vi "RampFunction.vi"(10 "Max Rate":dbl=1.0, 11 "Input":dbl(slide) scale=0.0..10.0) -> (3 "Output":dbl)   [LabVIEW 2016]
panel:
  # "r"
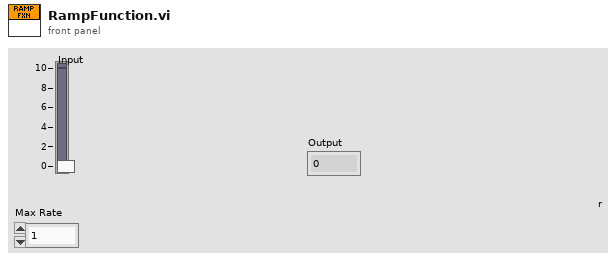
[diagram p1: front panel]
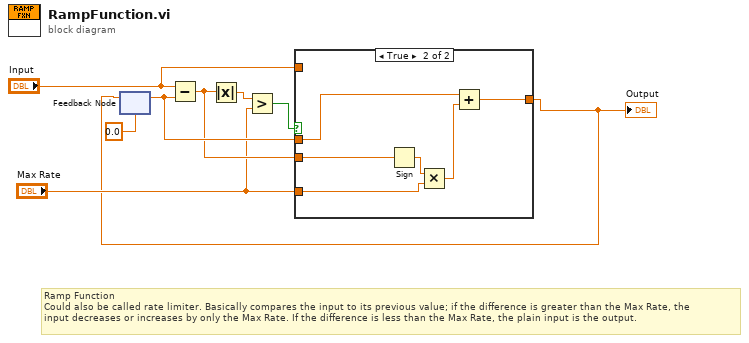
[diagram p0: block diagram]
diagram:
  # "Ramp Function\nCould also be called rate limiter. Basically compares the input to its previous value; if the difference is greater than the Max Rate, the \ninput decreases or increases by only the Max Rate. If the difference is less than the Max Rate, the plain input is the output."
  n1 = feedback #1(0.0 ("Input")) -> (w6:dbl)
  n2 = Subtract(x="Input", y=w6) -> (x-y=w5:dbl)
  n3 = Absolute Value(x=w5) -> (abs(x)=w8:dbl)
  n4 = Greater?(x=w8, y="Max Rate") -> (0:w7:bool)
  n5 = case shown="True" w7 {
    tunnel: w6 -> [_ w15]
    tunnel: w5 -> [_ w14]
    tunnel: "Max Rate" -> [_ w12]
    tunnel: [w9 w10] -> w1
    tunnel: "Input" -> [w9 _]
    frame False {
    }
    frame True {
      n6 = Sign(1:w14) -> (0:w13:dbl)
      n7 = Multiply(x=w13, y=w12) -> (x*y=w11:dbl)
      n8 = Add(x=w15, y=w11) -> (x+y=w10:dbl)
    }
  }
  "Output" <- w1
  n9 = feedback-in #1(w1) -> ()
